vi "HeaderTrap.vi"(0 "Index In":dbl=1.0, 1 "File Info":dbl[](array[numeric]), 2 "BD Frqs":dbl[](array[numeric]), 3 "Scan Data":dbl[](array[numeric]), 5 "Comment":string="testing confocal setup") -> (14 "Index Out":dbl, 15 "Trap Path":path, 16 "Trap File Out":refnum<file>)   [LabVIEW 2013]
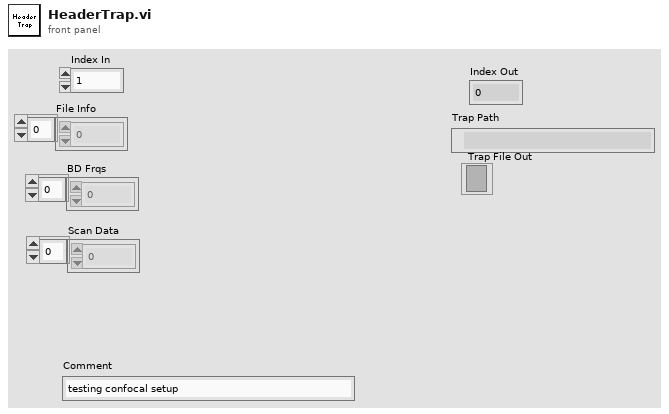
[diagram p1: front panel]
types:
  T1 = enum16{"big-endian, network order", "native, host order", "little-endian"}
  T2 = enum16{"open", "replace", "create", "open or create", "replace or create", "replace or create with confirmation"}
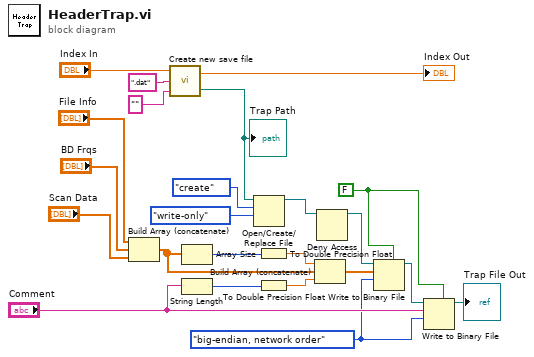
[diagram p0: block diagram]
diagram:
  w6 = FALSE ("prepend array or string size? (T)")
  w4 = T1."big-endian, network order" ("byte order (0:big-endian, network order)")
  n1 = Build Array (concatenate)("File Info", "BD Frqs", "Scan Data") -> (w23:dbl[])
  n2 = call "Create new save file.vi"("Insert"="", "Ext"=".dat", "Index In"="Index In") -> ("Path Out"=w19:path, "Index Out"=→"Index Out":dbl)
  "Trap Path" <- w19
  n3 = Array Size(array=w23) -> (size(s)=w12:i32)
  n4 = String Length(string="Comment") -> (length=w9:i32)
  n5 = Open/Create/Replace File(file path (use dialog)=w19, operation (0:open)=T2."create", access (0:read/write)=enum16{"read/write", "read-only", "write-only"}."write-only") -> (refnum out=w14:refnum<file>)  [unwired: 1 in, 4 out]
  n6 = To Double Precision Float(number=w12) -> (double precision float=w11:dbl)
  n7 = To Double Precision Float(number=w9) -> (double precision float=w8:dbl)
  n8 = Build Array (concatenate)(w11, w23, w8) -> (w10:dbl[])
  n9 = Deny Access(7:w14) -> (3:w13:refnum<file>)  [unwired: 1 in, 2 out]
  n10 = Write to Binary File(file (use dialog)=w13, data=w10, 5:w6, 9:w4) -> (refnum out=w7:refnum<file>)  [unwired: 1 in, 3 out]
  n11 = Write to Binary File(file (use dialog)=w7, data="Comment", 5:w6, 9:w4) -> (refnum out=→"Trap File Out":refnum<file>)  [unwired: 1 in, 3 out]
